vi "Start Sync.vi"(8 "error in (no error)":errorcluster, 11 "gRPC Server in":refnum<class "GreeterService.lvclass">) -> (0 "error out":errorcluster, 3 "gRPC Server out":refnum<class "GreeterService.lvclass">)   [LabVIEW 2019, in "Generated_server.lvlib" / "GreeterService.lvclass"]
uses:
  GreeterService.lvclass
  GreeterService.lvclass/GreeterService.ctl
  RPC Messages/Greeter_res.ctl
  RPC Messages/Greeter_res_res_oneof/Greeter_res_res_oneof.lvclass
  RPC Messages/Greeter_req_req_oneof/Greeter_req_req_oneof.lvclass/Greeter_req_req_oneof.ctl
  RPC Messages/Greeter_res_res_oneof/Greeter_res_res_oneof.lvclass/Greeter_res_res_oneof.ctl
  Generated_server.lvlib
  RPC Messages/Greeter_req_req_oneof/Greeter_req_req_oneof.lvclass
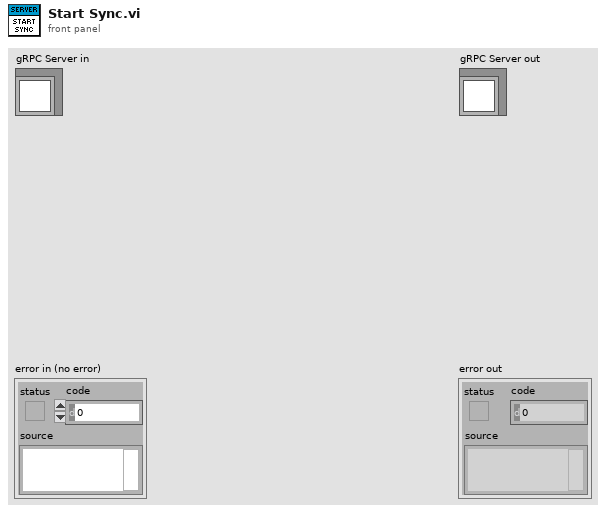
[diagram p1: front panel]
types:
  T1 = typedef "Generated_server.lvlib/GreeterService.lvclass/Server Internal UEs.ctl" = cluster{"GreeterService GetFeature Internal UE":refnum<user-event>}
  T2 = typedef "Generated_server.lvlib/GreeterService.lvclass/Server gRPC UEs.ctl" = cluster{"GreeterService GetFeature gRPC UE":refnum<user-event>}
  T3 = typedef "Generated_server.lvlib/Greeter_res.ctl" = cluster{"res_latitude":i32, "Greeter_res_res_oneof":refnum<class "Greeter_res_res_oneof.lvclass">}
  T4 = typedef "grpc-lvsupport-release.lvlib/grpcId.ctl" = u64
  T5 = typedef "Generated_server.lvlib/Greeter_req.ctl" = cluster{"req_latitude":i32, "Greeter_req_req_oneof":refnum<class "Greeter_req_req_oneof.lvclass">}
  T6 = typedef "grpc-lvsupport.lvlib/grpcId.ctl" = u64
  T7 = typedef "Generated_server.lvlib/Greeter_Color.ctl" = enum32{"RED", "GREEN", "BLUE"}
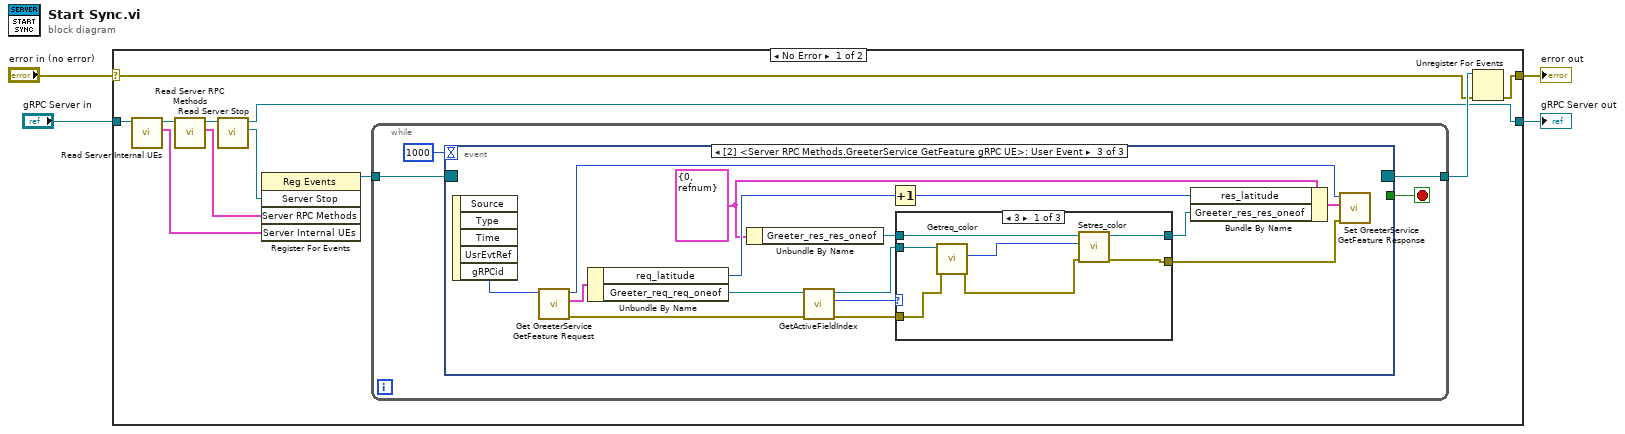
[diagram p0: block diagram]
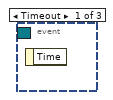
[diagram p2: hidden frame]
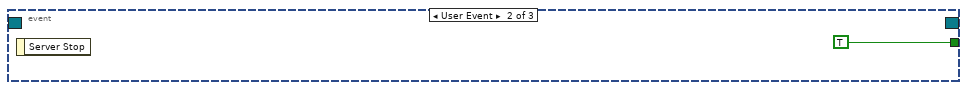
[diagram p3: hidden frame]
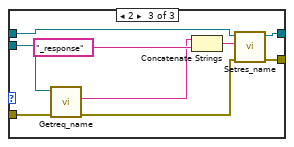
[diagram p5: hidden frame]
diagram:
  n1 = case shown="No Error" "error in (no error)" {
    selector: "error in (no error)" -> [w9 w55]
    tunnel: [w8 w55] -> w3
    tunnel: [w6 w54] -> w1
    tunnel: "gRPC Server in" -> [w15 w54]
    frame No Error {
      n2 = call "Read Server Internal UEs.vi"("SignalGeneratorService in"=w15) -> ("Server Internal UEs"=w13:T1, "SignalGeneratorService out"=w14:refnum<class "GreeterService.lvclass">)  [unwired: 8 in, 1 out]
      n3 = call "Read Server RPC Methods.vi"("SignalGeneratorService in"=w14) -> ("Server RPC Methods"=w7:T2, "SignalGeneratorService out"=w12:refnum<class "GreeterService.lvclass">)  [unwired: 8 in, 1 out]
      n4 = call-dynamic "Read Server Stop.vi"("iService in"=w12) -> ("Server Stop"=w5:refnum<user-event>, "iService out"=w6:refnum<class "GreeterService.lvclass">)  [unwired: 8 in, 1 out]
      n5 = register-events(w5, w7, w13) -> (reference out=w11:refnum<event-registration>)  [unwired: 2 in, 1 out]
      n6 = while {
        tunnel: w11 -> [w19]
        tunnel: [w17] -> w10
        stop <- w18 stop-if-true
        n7 = event "RPC Methods Event Structure" shown="[2] <Server RPC Methods.GreeterService GetFeature gRPC UE>: User Event" {
          selector: w19 -> [_ _ _]
          dyn-events: [_ _ _] -> w17
          timeout: 1000 -> [_ _ _]
          tunnel: [_ TRUE _] -> w18
          event Timeout {
            n8 = event-data() -> ()  [unwired: 1 in, 1 out]
          }
          event User Event {
            n9 = event-data() -> ()  [unwired: 1 in, 1 out]
          }
          event User Event {
            w24 = T3 {"res_latitude"=0, "Greeter_res_res_oneof"=refnum} ("Message Data")
            n10 = event-data() -> ("gRPCid"=w35:T4)  [unwired: 1 in, 4 out]
            n11 = call "Get GreeterService GetFeature Request.vi"("gRPCid in"=w35) -> ("error out"=w26:errorcluster, "Message Data"=w34:T5, "gRPCid out"=w21:T6)  [unwired: 8 in]
            n12 = Unbundle By Name(w34) -> ("req_latitude"=w33:i32, "Greeter_req_req_oneof"=w31:refnum<class "Greeter_req_req_oneof.lvclass">)
            n13 = Unbundle By Name(w24) -> ("Greeter_res_res_oneof"=w29:refnum<class "Greeter_res_res_oneof.lvclass">)
            n14 = call "GetActiveFieldIndex.vi"("error in (no error)"=w26, "OneOfTemplate in"=w31) -> ("error out"=w27:errorcluster, "Active Field Index"=w30:i32, "OneOfTemplate out"=w28:refnum<class "Greeter_req_req_oneof.lvclass">)  [unwired: 7 in]
            n15 = Increment(x=w33) -> (x+1=w32:i32)
            n16 = case shown="3" w30 {
              tunnel: w29 -> [w39 w44 w47]
              tunnel: w28 -> [w41 _ w53]
              tunnel: w27 -> [w42 w43 w52]
              tunnel: [w38 w44 w46] -> w25
              tunnel: [w37 w43 w45] -> w22
              frame 3 {
                n17 = call "Getreq_color.vi"("error in (no error)"=w42, "OneOfTemplate in"=w41) -> ("error out"=w40:errorcluster, "Get_Val"=w36:T7)  [unwired: 7 in, 1 out]
                n18 = call "Setres_color.vi"("error in (no error)"=w40, "Set_Val"=w36, "OneOfTemplate in"=w39) -> ("error out"=w37:errorcluster, "OneOfTemplate out"=w38:refnum<class "Greeter_res_res_oneof.lvclass">)  [unwired: 7 in]
              }
              frame Default {
              }
              frame 2 {
                n19 = call "Getreq_name.vi"("error in (no error)"=w52, "OneOfTemplate in"=w53) -> ("error out"=w51:errorcluster, "Get_Val"=w49:string)  [unwired: 7 in, 1 out]
                n20 = Concatenate Strings(w49, "_response" ("string")) -> (w48:string)
                n21 = call "Setres_name.vi"("error in (no error)"=w51, "Set_Val"=w48, "OneOfTemplate in"=w47) -> ("error out"=w45:errorcluster, "OneOfTemplate out"=w46:refnum<class "Greeter_res_res_oneof.lvclass">)  [unwired: 7 in]
              }
            }
            n22 = Bundle By Name(cluster=w24, "res_latitude"=w32, "Greeter_res_res_oneof"=w25) -> (w23:T3)
            n23 = call "Set GreeterService GetFeature Response.vi"("error in (no error)"=w22, "Message Data"=w23, "gRPCid in"=w21) -> ()  [unwired: 8 in, 1 out]
          }
        }
      }
      n24 = Unregister For Events(event registration refnum=w10, error in=w9) -> (error out=w8:errorcluster)
    }
    frame Error {
    }
  }
  "error out" <- w3
  "gRPC Server out" <- w1
